vi "GetInspectionResults.vi"(6 "Select Inspection":T1, 7 "Image Step Name (default last image used by inspection)":cluster{"State Name":string, "Step Name":string}={"State Name"="Variable", "Step Name"="IMG_CameraAcquisition"}, 8 "error in (no error)":errorcluster, 9 "StepName":string, 10 "Image Enable":bool, 11 "Refnum in":T3) -> (0 "error out":errorcluster, 1 "Results":T2, 2 "Image Dst Out":T4, 3 "Refnum out":T3, 5 "Inspection Status":bool)   [LabVIEW 2014]
uses:
  <vilib>/vision/Image Controls.llb/IMAQ Image.ctl
  <vilib>/userdefined/High Color/VBAIInterface.ctl
  c_VBAI_SelcectInspection.ctl
  <vilib>/vision/Vision Builder AI/API.llb/IVB Interface - Set Variable Mode.ctl
  <vilib>/vision/Vision Builder AI/API.llb/VBAI Interface - Get Inspection Image (By Name).vi
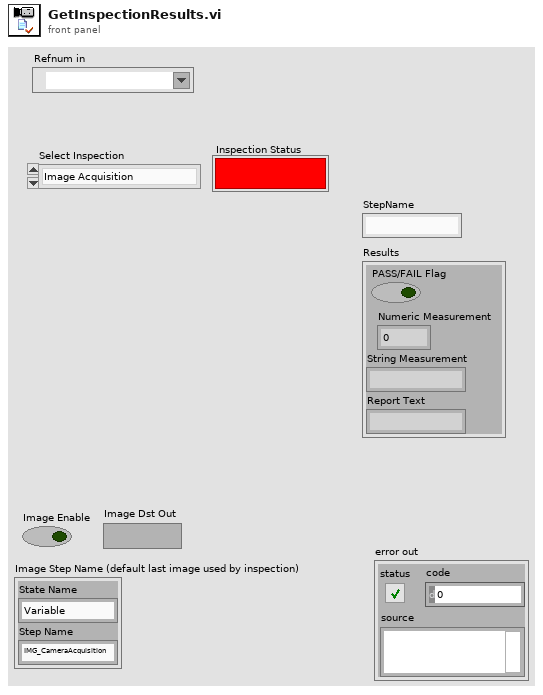
[diagram p1: front panel]
types:
  T1 = typedef "c_VBAI_SelcectInspection.ctl" = enum16{"Image Acquisition", "Find Reference", "Chip Alignment", "Adjustment", "Porbecard Positioning"}
  T2 = cluster{"PASS/FAIL Flag":bool, "Numeric Measurement":dbl, "String Measurement":string, "Report Text":string}
  T3 = typedef "VBAIInterface.ctl" = refnum<k21>
  T4 = typedef "IMAQ Image.ctl" = refnum<image>
  T5 = typedef "IVB Interface - Set Variable Mode.ctl" = enum16{"Update on Next Iteration", "Update Immediately"}
  T6 = typedef "IVB Interface - Step Info.ctl" = cluster{"State Name":string, "Step Name":string, "Step GUID":string, "Process Class":string, "Pass/Fail Conditions Data":cluster{"Condition Type":enum16{"Numeric Condition", "String Condition"}, "Numeric Condition":cluster{"Used":bool, "Value 1":dbl, "Value 2":dbl, "Function":enum16{"Less", "Less or Equal", "Greater", "Greater or Equal", "In Range", "Equal", "Not Equal"}}, "String Condition":cluster{"Used":bool, "Value 1":string, "Value 2":string, "Function":enum16{"Equal", "Not equal", "Match Pattern", "Less", "Less or Equal", "Greater", "Greater or Equal", "In Range"}}}[]}
  T7 = cluster{"PASS/FAIL Flag":bool, "Numeric Measurement":dbl, "String Measurement":string, "Report Text":string}[]
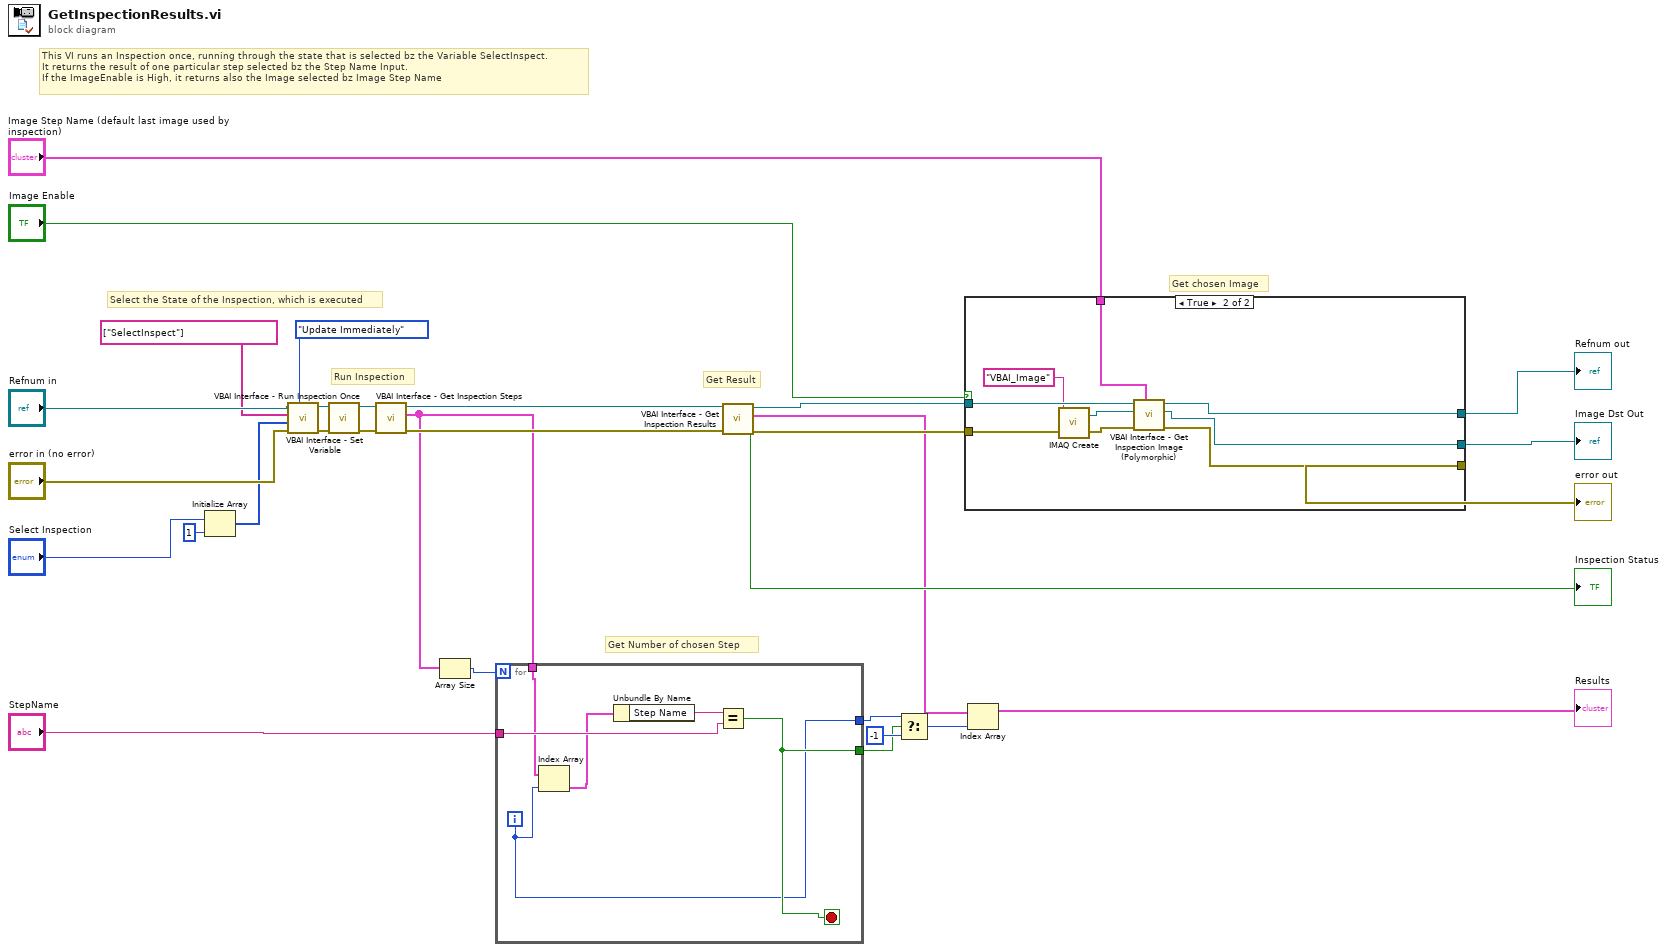
[diagram p0: block diagram]
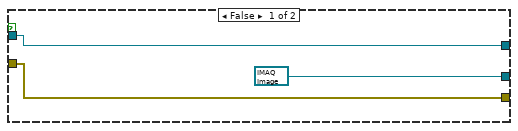
[diagram p2: hidden frame]
diagram:
  # "Select the State of the Inspection, which is executed"
  # "This VI runs an Inspection once, running through the state that is selected bz the Variable SelectInspect. \nIt returns the result of one particular step selected bz the Step Name Input.\nIf the ImageEnable is High, it returns also the Image selected bz Image Step Name"
  # "Get chosen Image"
  # "Get Result"
  # "Get Number of chosen Step"
  # "Run Inspection"
  n1 = Initialize Array("Select Inspection", 1 ("dimension size")) -> (w3:T1[])
  n2 = call <vilib>:"VBAI Interface - Set Variable.vi"("Mode"=IVB_Interface_-_Set_Variable_Mode."Update Immediately", "error in"="error in (no error)", "Variable Values"=w3, "Variable Names"=string[] ["SelectInspect"], "Session In"="Refnum in") -> ("error out"=w1:errorcluster, "Session Out"=w8:T3)  [unwired: 5 in]
  n3 = call <vilib>:"VBAI Interface - Run Inspection Once.vi"("error in"=w1, "Session In"=w8) -> ("error out"=w19:errorcluster, "Session Out"=w20:T3)  [unwired: 8 in]
  n4 = call <vilib>:"VBAI Interface - Get Inspection Steps.vi"("error in"=w19, "Session In"=w20) -> ("error out"=w17:errorcluster, "Inspection Steps"=w14:T6[], "Session Out"=w18:T3)  [unwired: 6 in, 1 out]
  n5 = Array Size(array=w14) -> (size(s)=w15:i32)
  n6 = for {
    N: w15 -> [_]
    tunnel: w14 -> [w31]
    tunnel: "StepName" -> [w36]
    tunnel: [w32] -> w13
    tunnel: [w35] -> w11
    i -> [w32]
    stop <- w35 stop-if-true
    n7 = Index Array(array=w31, index=w32) -> (element=w33:T6)
    n8 = Unbundle By Name(w33) -> ("Step Name"=w34:string)
    n9 = Equal?(x=w34, y=w36) -> (x = y?=w35:bool)
  }
  n10 = call <vilib>:"VBAI Interface - Get Inspection Results.vi"("error in"=w17, "Session In"=w18) -> ("error out"=w25:errorcluster, "Inspection Status"=→"Inspection Status":bool, "Step Results"=w21:T7, "Session Out"=w24:T3)  [unwired: 3 in, 3 out]
  n11 = Select(t=w13, s=w11, f=-1) -> (s? t:f=w10:i32)
  n12 = case shown="True" "Image Enable" {
    tunnel: w24 -> [w39 w48]
    tunnel: w25 -> [w38 w45]
    tunnel: [w39 w43] -> w27
    tunnel: [w38 w42] -> w28
    tunnel: [T4 refnum ("Image Dst Out") w41] -> w29
    tunnel: "Image Step Name (default last image used by inspection)" -> [_ w40]
    frame False {
    }
    frame True {
      n13 = call "IMAQ Create"("Image Name"="VBAI_Image", "error in (no error)"=w45) -> ("New Image"=w47:T4, "error out"=w46:errorcluster)  [unwired: 3 in]
      n14 = call-poly <vilib>:"VBAI Interface - Get Inspection Image (Polymorphic).vi"("Image Step Name (default last image used by inspection)"=w40, "error in"=w46, "Image Dest"=w47, "Session In"=w48) -> ("error out"=w42:errorcluster, "Image Dst Out"=w41:T4, "Session Out"=w43:T3)  [unwired: 4 in, 1 out]
    }
  }
  "Image Dst Out" <- w29
  "error out" <- w28
  "Refnum out" <- w27
  n15 = Index Array(array=w21, index=w10) -> (element=→"Results":T2)
